vi "Split Images_Vision Task.vi"() -> (2 "error out":errorcluster, 3 "Extracted Section":T1(plugin-control))   [LabVIEW 2020]
doc: "This VI demonstrates how to use the functions from the Vision Development Module (VDM) to continuously split an image into sections.\nYou can specify the size of a section (X Step Size and Y Step Size). The VI will calculate the number of sections in the image and will extract section after section from the image."
uses:
  <vilib>/vision/NI_Vision_Development_Module.lvlib
  <vilib>/ptbypt/NI_PtbyPt.lvlib
panel:
  out "Mean Value of Ry for entire surface":dbl format="%0.2f"
  out "Current Queue":dbl[](array[numeric])
  out "Mean Value of Ry for each sections":dbl format="%0.2f"
  in  "stop":bool
  out "Segmenting  Image":T1(plugin-control)
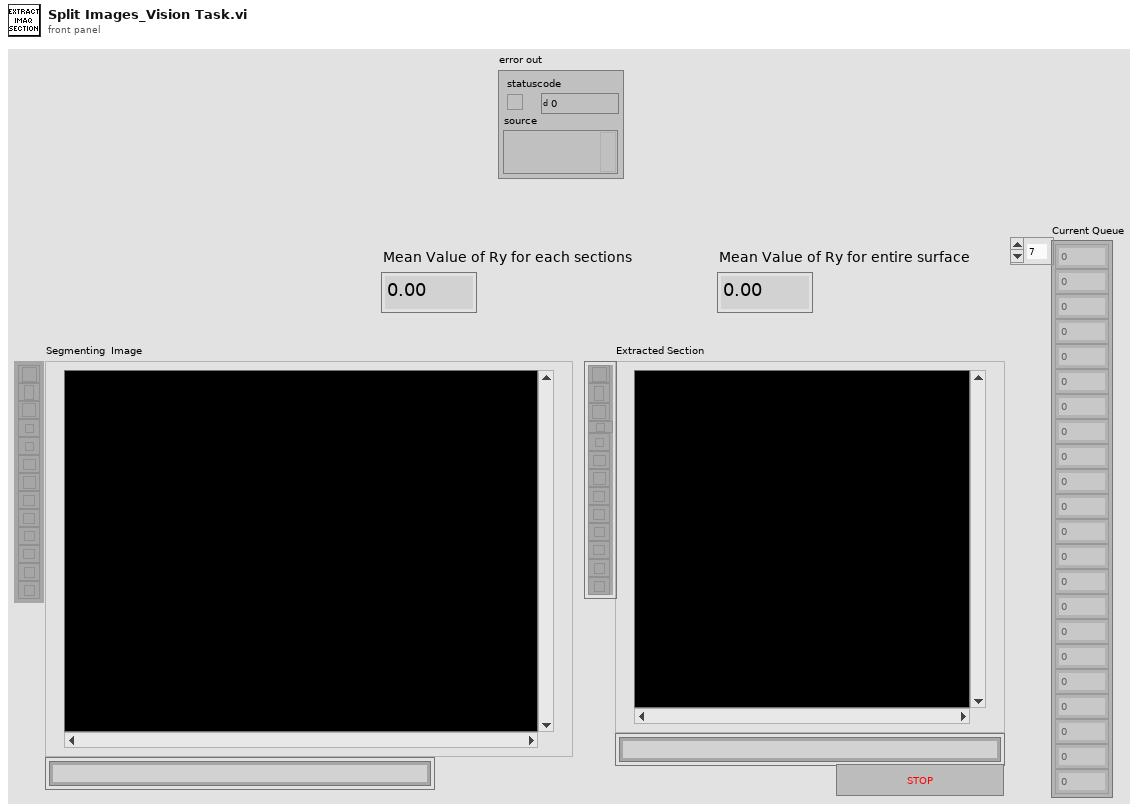
[diagram p1: front panel]
types:
  T1 = typedef "IMAQ Image.ctl" = refnum<image>
  T2 = typedef "Image Type" = u32
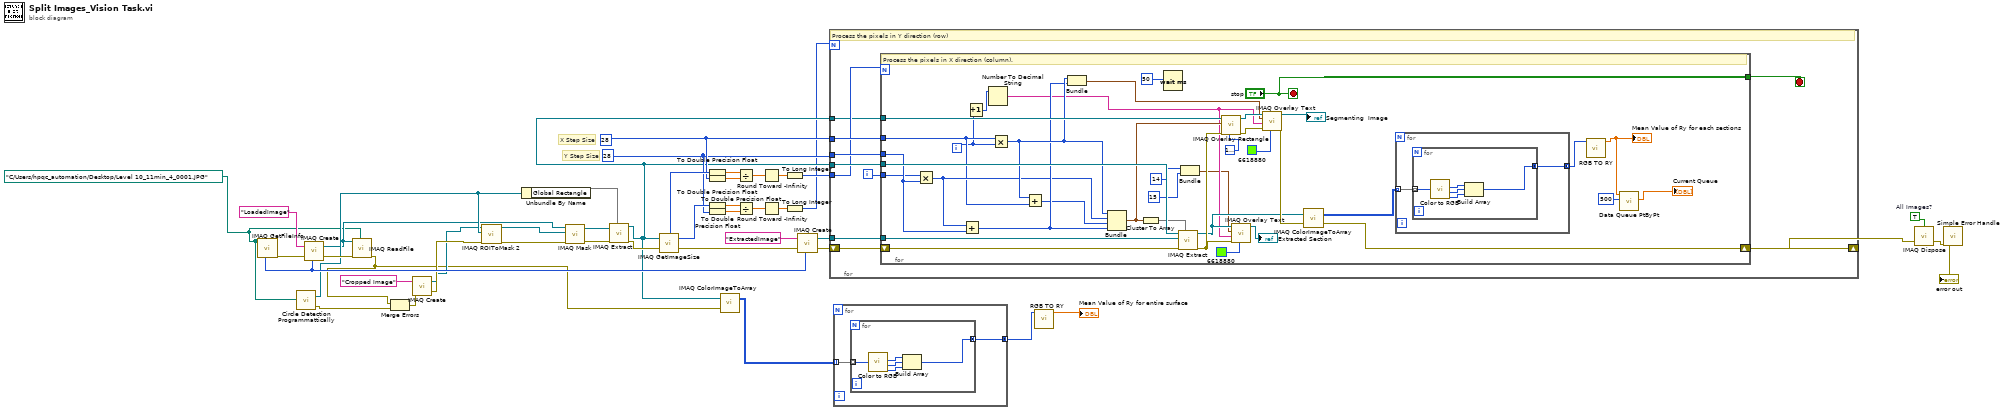
[diagram p0: block diagram]
diagram:
  w1 = path "C:/Users/hpqc_automation/Desktop/Level 10_11min_4_0001.JPG" ("File Path")
  w22 = 28 ("X Step Size (Pixel)")
  w24 = 28 ("X Step Size (Pixel)")
  w40 = TRUE  # All Images?
  # "Y Step Size"
  # "X Step Size"
  n1 = call "IMAQ GetFileInfo"("File Path"=w1) -> ("error out"=w29:errorcluster, "Image Type"=w26:T2)  [unwired: 4 in, 5 out]
  n2 = call "Circle Detection Programmattically.vi"("File Path"=w1) -> ("Image Out"=w13:T1, "error out"=w20:errorcluster)  [unwired: 23 in, 2 out]
  n3 = call "IMAQ Create"("Image Name"="LoadedImage", "Image Type"=w26, "error in (no error)"=w29) -> ("New Image"=w12:T1, "error out"=w44:errorcluster)  [unwired: 1 in, 1 out]
  n4 = call "IMAQ ReadFile"("File Path"=w1, "error in (no error)"=w44, "Image"=w12) -> ("error out"=w4:errorcluster)  [unwired: 2 in, 6 out]
  n5 = Merge Errors(w4, w20) -> (w19:errorcluster)
  n6 = call "IMAQ Create"("Image Name"="Cropped Image", "error in (no error)"=w19) -> ("New Image"=w10:T1, "error out"=w11:errorcluster)  [unwired: 3 in]
  n7 = call "IMAQ ROIToMask 2"("error in (no error)"=w11, "ROI Descriptor"=w13, "Image"=w10) -> ("error out"=w15:errorcluster, "Image Out"=w18:T1)  [unwired: 6 in, 1 out]
  n8 = Unbundle By Name(w13) -> ("Global Rectangle"=w14)
  n9 = call "IMAQ Mask"("error in (no error)"=w15, "Image Mask"=w18, "Image Src"=w12) -> ("error out"=w16:errorcluster, "Image Dst Out"=w17:T1)  [unwired: 2 in]
  n10 = call "IMAQ Extract"("Optional Rectangle"=w14, "error in (no error)"=w16, "Image Src"=w17) -> ("error out"=w8:errorcluster, "Image Dst Out"=w3:T1)  [unwired: 7 in]
  n11 = call "IMAQ GetImageSize"("Image"=w3, "error in (no error)"=w8) -> ("Y Resolution"=w31:i32, "X Resolution"=w33:i32, "error out"=w38:errorcluster)  [unwired: 2 out]
  n12 = To Double Precision Float(number=w33) -> (double precision float=w32:dbl)
  n13 = To Double Precision Float(number=w24) -> (double precision float=w27:dbl)
  n14 = To Double Precision Float(number=w31) -> (double precision float=w30:dbl)
  n15 = To Double Precision Float(number=w22) -> (double precision float=w28:dbl)
  n16 = call "IMAQ ColorImageToArray"("Image"=w3, "error in (no error)"=w4) -> ("Image Pixels (U32)"=w7:u32[][])  [unwired: 2 in, 2 out]
  n17 = Divide(x=w32, y=w27) -> (x/y=w37:dbl)
  n18 = Divide(x=w30, y=w28) -> (x/y=w35:dbl)
  n19 = Round Toward -Infinity(1:w37) -> (0:w36:dbl)
  n20 = Round Toward -Infinity(1:w35) -> (0:w34:dbl)
  n21 = To Long Integer(number=w36) -> (32bit integer=w23:i32)
  n22 = To Long Integer(number=w34) -> (32bit integer=w2:i32)
  n23 = call "IMAQ Create"("Image Name"="ExtractedImage", "Image Type"=w26, "error in (no error)"=w38) -> ("New Image"=w42:T1, "error out"=w39:errorcluster)  [unwired: 1 in, 1 out]
  n24 = for {
    N: w2 -> [_]
    tunnel: w3 -> [w54]
    tunnel: w42 -> [w53]
    tunnel: w23 -> [w46]
    shift-right: [w52] -> w9
    shift-left: w39 -> [w51]
    tunnel: w24 -> [w48]
    tunnel: w22 -> [w47]
    tunnel: w3 -> [w45]
    i -> [w50]
    stop <- w49 stop-if-true
    # "Process the pixels in Y direction (row)"
    n25 = for {
      N: w46 -> [_]
      tunnel: w54 -> [w91]
      tunnel: w53 -> [w92]
      tunnel: w50 -> [w63]
      tunnel: ["stop"] -> w49
      shift-right: [w82] -> w52
      shift-left: w51 -> [w90]
      tunnel: w48 -> [w57]
      tunnel: w47 -> [w88]
      tunnel: w45 -> [w87]
      i -> [w56]
      stop <- "stop" stop-if-true
      # "Process the pixels in X direction (column)."
      n26 = Multiply(x=w63, y=w88) -> (x*y=w62:i32)
      n27 = Add(x=w62, y=w88) -> (x+y=w71:i32)
      n28 = Increment(x=w56) -> (x+1=w55:i32)
      n29 = Number To Decimal String(number=w55) -> (decimal integer string=w64:string)  [unwired: 1 in]
      n30 = Multiply(x=w57, y=w56) -> (x*y=w72:i32)
      n31 = Add(x=w72, y=w57) -> (x+y=w61:i32)
      n32 = Bundle(w72, w71) -> (w66:cluster{i32, i32})  [unwired: 1 in]
      n33 = Bundle(w72, w62, w61, w71) -> (w86:cluster{i32, i32, i32, i32})  [unwired: 1 in]
      n34 = Cluster To Array(cluster=w86) -> (array=w85:i32[])
      n35 = Wait (ms)(milliseconds to wait=u32 50 ("Wait time (ms) between frames")) -> ()  [unwired: 1 out]
      n36 = call "IMAQ Extract"("Optional Rectangle"=w85, "error in (no error)"=w90, "Image Dst"=w92, "Image Src"=w91) -> ("error out"=w68:errorcluster, "Image Dst Out"=w67:T1)  [unwired: 2 in, 4 out]
      n37 = Bundle(14, 15) -> (w60:cluster{i32, i32})  [unwired: 1 in]
      n38 = call "IMAQ Overlay Rectangle"("Color"=u32 16777222, "error in (no error)"=w68, "Rectangle"=w86, "Image"=w87) -> ("error out"=w76:errorcluster, "Image Out"=w74:T1)  [unwired: 6 in]
      n39 = call "IMAQ Overlay Text"("Text Color (black)"=u32 6618880 ("Color"), "error in (no error)"=w68, "String"=w64, "Origin"=w60, "Image"=w67) -> ("Image Out"=→"Extracted Section":T1)  [unwired: 5 in, 1 out]
      n40 = call "IMAQ Overlay Text"("Text Color (black)"=u32 6618880 ("Color"), "error in (no error)"=w76, "String"=w64, "Origin"=w66, "Image"=w74) -> ("error out"=w75:errorcluster, "Image Out"=→"Segmenting  Image":T1)  [unwired: 5 in]
      n41 = call "IMAQ ColorImageToArray"("Image"=w67, "error in (no error)"=w75) -> ("Image Pixels (U32)"=w81:u32[][], "error out"=w82:errorcluster)  [unwired: 2 in, 1 out]
      n42 = for {
        tunnel: w81 -> [w94] mode=indexing
        tunnel: [w93] -> w80 mode=concatenating
        n43 = for {
          tunnel: w94 -> [w99] mode=indexing
          tunnel: [w98] -> w93 mode=concatenating
          n44 = call <vilib>:"Color to RGB.vi"("Color"=w99) -> ("R"=w97:u8, "G"=w96:u8, "B"=w95:u8)  [unwired: 1 out]
          n45 = Build Array(w97, w96, w95) -> (w98:u8[])
        }
      }
      n46 = call "RGB TO RY.vi"("Array"=w80) -> ("Mean Value of Ry"=w78:dbl)  [unwired: 10 in]
      "Mean Value of Ry for each sections" <- w78
      n47 = call <vilib>:"Data Queue PtByPt.vi"("sample length"=500, "input data point"=w78) -> ("Current Queue"=→"Current Queue":dbl[])  [unwired: 5 in, 4 out]
    }
  }
  n48 = for {
    tunnel: w7 -> [w101] mode=indexing
    tunnel: [w100] -> w6 mode=concatenating
    n49 = for {
      tunnel: w101 -> [w106] mode=indexing
      tunnel: [w105] -> w100 mode=concatenating
      n50 = call <vilib>:"Color to RGB.vi"("Color"=w106) -> ("R"=w104:u8, "G"=w103:u8, "B"=w102:u8)  [unwired: 1 out]
      n51 = Build Array(w104, w103, w102) -> (w105:u8[])
    }
  }
  n52 = call "RGB TO RY.vi"("Array"=w6) -> ("Mean Value of Ry"=→"Mean Value of Ry for entire surface":dbl)  [unwired: 10 in]
  n53 = call "IMAQ Dispose"("All Images? (No)"=w40, "error in (no error)"=w9) -> ("error out"=w25:errorcluster)  [unwired: 1 in, 3 out]
  "error out" <- w25
  n54 = call <vilib>:"Simple Error Handler.vi"("error in (no error)"=w25) -> ()  [unwired: 1 in, 8 out]
